vi "N6701A_WaitforPowerDown.vi"(5 "Timeout (s)":dbl, 7 "Current Threshold (A)":dbl, 8 "error in (no error)":errorcluster, 10 "Channel Name (1)":string="2", 11 "VISA resource name":refnum<visa-resource-name>="PS2") -> (0 "error out":errorcluster)   [LabVIEW 2015]
uses:
  <instrlib>/Agilent N6700 Series/Agilent N6700 Series.lvlib
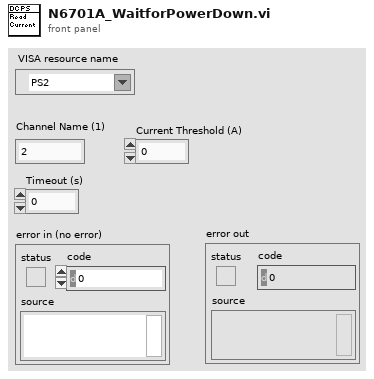
[diagram p1: front panel]
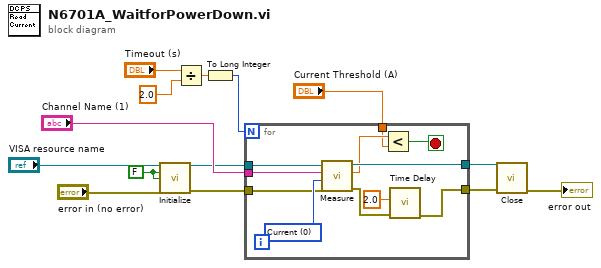
[diagram p0: block diagram]
diagram:
  w11 = FALSE ("ID Query? (T: Yes)")
  n1 = call <instrlib>:"Initialize.vi"("VISA resource name"="VISA resource name", "ID Query? (T: Yes)"=w11, "Reset? (T: Yes)"=w11, "error in (no error)"="error in (no error)") -> ("VISA resource name out"=w10:refnum<visa-resource-name>, "error out"=w9:errorcluster)  [unwired: 10 in]
  n2 = Divide(x="Timeout (s)", y=2.0) -> (x/y=w5:dbl)
  n3 = To Long Integer(number=w5) -> (32bit integer=w4:i32)
  n4 = for {
    N: w4 -> [_]
    tunnel: "Channel Name (1)" -> [w24]
    tunnel: w10 -> [w23]
    tunnel: w9 -> [w22]
    tunnel: [w19] -> w2
    tunnel: [w18] -> w3
    tunnel: "Current Threshold (A)" -> [w16]
    stop <- w15 stop-if-true
    w25 = 0 items=["Voltage"=1, "Current"=0] ("Measurement Type (1: Voltage)")
    n5 = call <instrlib>:"Measure.vi"("error in (no error)"=w22, "Measurement Type (1: Voltage)"=w25, "Channel Name (1)"=w24, "VISA resource name"=w23) -> ("error out"=w21:errorcluster, "Measurement"=w17:dbl, "VISA resource name out"=w18:refnum<visa-resource-name>)  [unwired: 5 in]
    n6 = Less?(x=w17, y=w16) -> (x < y?=w15:bool)
    n7 = call "Time Delay"("error in (no error)"=w21, "Delay Time (s)"=2.0) -> ("error out"=w19:errorcluster)  [unwired: 9 in]
  }
  n8 = call <instrlib>:"Close.vi"("VISA resource name"=w3, "error in (no error)"=w2) -> ("error out"=→"error out":errorcluster)  [unwired: 13 in]
